vi "TestXYRobot.vi"() -> ()   [LabVIEW 2012]
uses:
  XY Stage/XYStage.llb/GlobalXYStage.vi
panel:
  in  "robot limits":T1={"xmin"=-16850, "xmax"=-1660, "ymin"=-15485, "ymax"=-550}
  in  "Home":bool
  out "XY Graph":cluster{"Y":dbl[], "Y":dbl[]}[](graph)=[{"Y"=[-1660.0, -16850.0, -16850.0, -1660.0, -1660.0], "Y"=[-550.0, -550.0, -15485.0, -15485.0, -550.0]}]
  in  "plot buffer":i32=5
  in  "Motor acc":i32=500
  in  "Motor low speed":i32=100
  in  "Motor high speed":i32=5000
  in  "Robot Position":T2(radio)
  in  "stop":bool
  out "Y position":i32=-550
  out "X position":i32=-1660
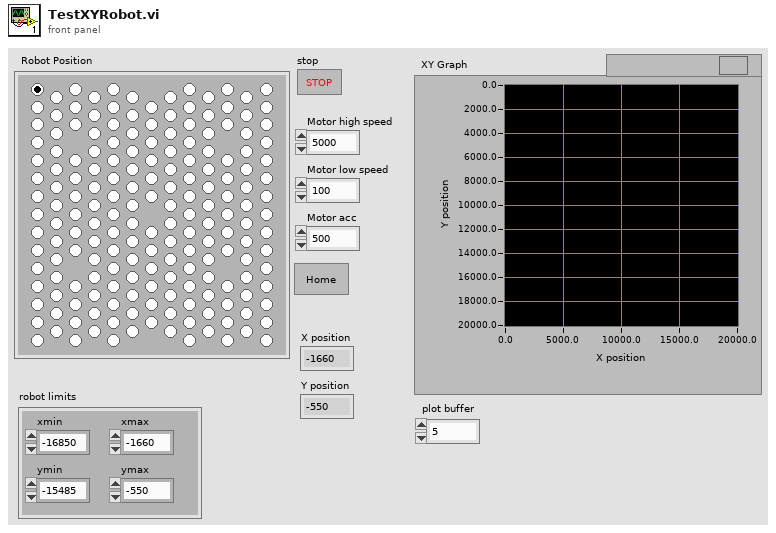
[diagram p1: front panel]
types:
  T1 = cluster{"xmin":i32, "xmax":i32, "ymin":i32, "ymax":i32}
  T2 = enum32{"Radio Selection 1", "Radio Selection 2", "Radio Selection 3", "Radio Selection 5", "Radio Selection 6", "Radio Selection 8", "Radio Selection 13", "Radio Selection 14", "Radio Selection 15", "Radio Selection 16", "Radio Selection 17", "Radio Selection 18", "Radio Selection 7", "Radio Selection 9", "Radio Selection 10", "Radio Selection 11", "Radio Selection 12", "Radio Selection 19", "Radio Selection 20", "Radio Selection 21", "Radio Selection 22", "Radio Selection 23", "Radio Selection 24", "Radio Selection 25", "Radio Selection 26", "Radio Selection 27", "Radio Selection 28", "Radio Selection 29", "Radio Selection 30", "Radio Selection 31", "Radio Selection 32", "Radio Selection 33", "Radio Selection 34", "Radio Selection 35", "Radio Selection 36", "Radio Selection 37", "Radio Selection 38", "Radio Selection 39", "Radio Selection 40", "Radio Selection 42", "Radio Selection 43", "Radio Selection 44", "Radio Selection 46", "Radio Selection 41", "Radio Selection 45", "Radio Selection 47", "Radio Selection 48", "Radio Selection 49", "Radio Selection 50", "Radio Selection 51", "Radio Selection 52", "Radio Selection 53", "Radio Selection 54", "Radio Selection 55", "Radio Selection 56", "Radio Selection 57", "Radio Selection 58", "Radio Selection 59", "Radio Selection 60", "Radio Selection 61", "Radio Selection 62", "Radio Selection 63", "Radio Selection 64", "Radio Selection 65", "Radio Selection 66", "Radio Selection 67", "Radio Selection 68", "Radio Selection 69", "Radio Selection 70", "Radio Selection 71", "Radio Selection 72", "Radio Selection 73", "Radio Selection 74", "Radio Selection 75", "Radio Selection 76", "Radio Selection 77", "Radio Selection 78", "Radio Selection 79", "Radio Selection 80", "Radio Selection 81", "Radio Selection 82", "Radio Selection 83", "Radio Selection 84", "Radio Selection 85", "Radio Selection 86", "Radio Selection 87", "Radio Selection 88", "Radio Selection 89", "Radio Selection 4", "Radio Selection 90", "Radio Selection 91", "Radio Selection 92", "Radio Selection 93", "Radio Selection 94", "Radio Selection 95", "Radio Selection 96", "Radio Selection 97", "Radio Selection 98", "Radio Selection 99", "Radio Selection 100", "Radio Selection 101", "Radio Selection 102", "Radio Selection 103", "Radio Selection 104", "Radio Selection 105", "Radio Selection 106", "Radio Selection 107", "Radio Selection 108", "Radio Selection 109", "Radio Selection 110", "Radio Selection 111", "Radio Selection 112", "Radio Selection 113", "Radio Selection 114", "Radio Selection 115", "Radio Selection 116", "Radio Selection 117", "Radio Selection 118", "Radio Selection 119", "Radio Selection 120", "Radio Selection 121", "Radio Selection 122", "Radio Selection 123", "Radio Selection 124", "Radio Selection 125", "Radio Selection 126", "Radio Selection 127", "Radio Selection 128", "Radio Selection 129", "Radio Selection 130", "Radio Selection 131", "Radio Selection 132", "Radio Selection 133", "Radio Selection 134", "Radio Selection 135", "Radio Selection 136", "Radio Selection 137", "Radio Selection 138", "Radio Selection 139", "Radio Selection 140", "Radio Selection 141", "Radio Selection 142", "Radio Selection 143", "Radio Selection 144", "Radio Selection 145", "Radio Selection 146", "Radio Selection 147", "Radio Selection 148", "Radio Selection 149", "Radio Selection 150", "Radio Selection 151", "Radio Selection 152", "Radio Selection 153", "Radio Selection 154", "Radio Selection 155", "Radio Selection 156", "Radio Selection 157", "Radio Selection 158", "Radio Selection 159", "Radio Selection 160", "Radio Selection 161", "Radio Selection 162", "Radio Selection 163", "Radio Selection 164", "Radio Selection 165", "Radio Selection 166", "Radio Selection 167", "Radio Selection 168", "Radio Selection 169", "Radio Selection 170", "Radio Selection 171", "Radio Selection 172", "Radio Selection 173", "Radio Selection 174", "Radio Selection 175", "Radio Selection 176", "Radio Selection 177", "Radio Selection 178", "Radio Selection 179", "Radio Selection 180", "Radio Selection 181", "Radio Selection 182"}
  T3 = enum8{"Enabled", "Disabled", "Disabled and Grayed Out"}
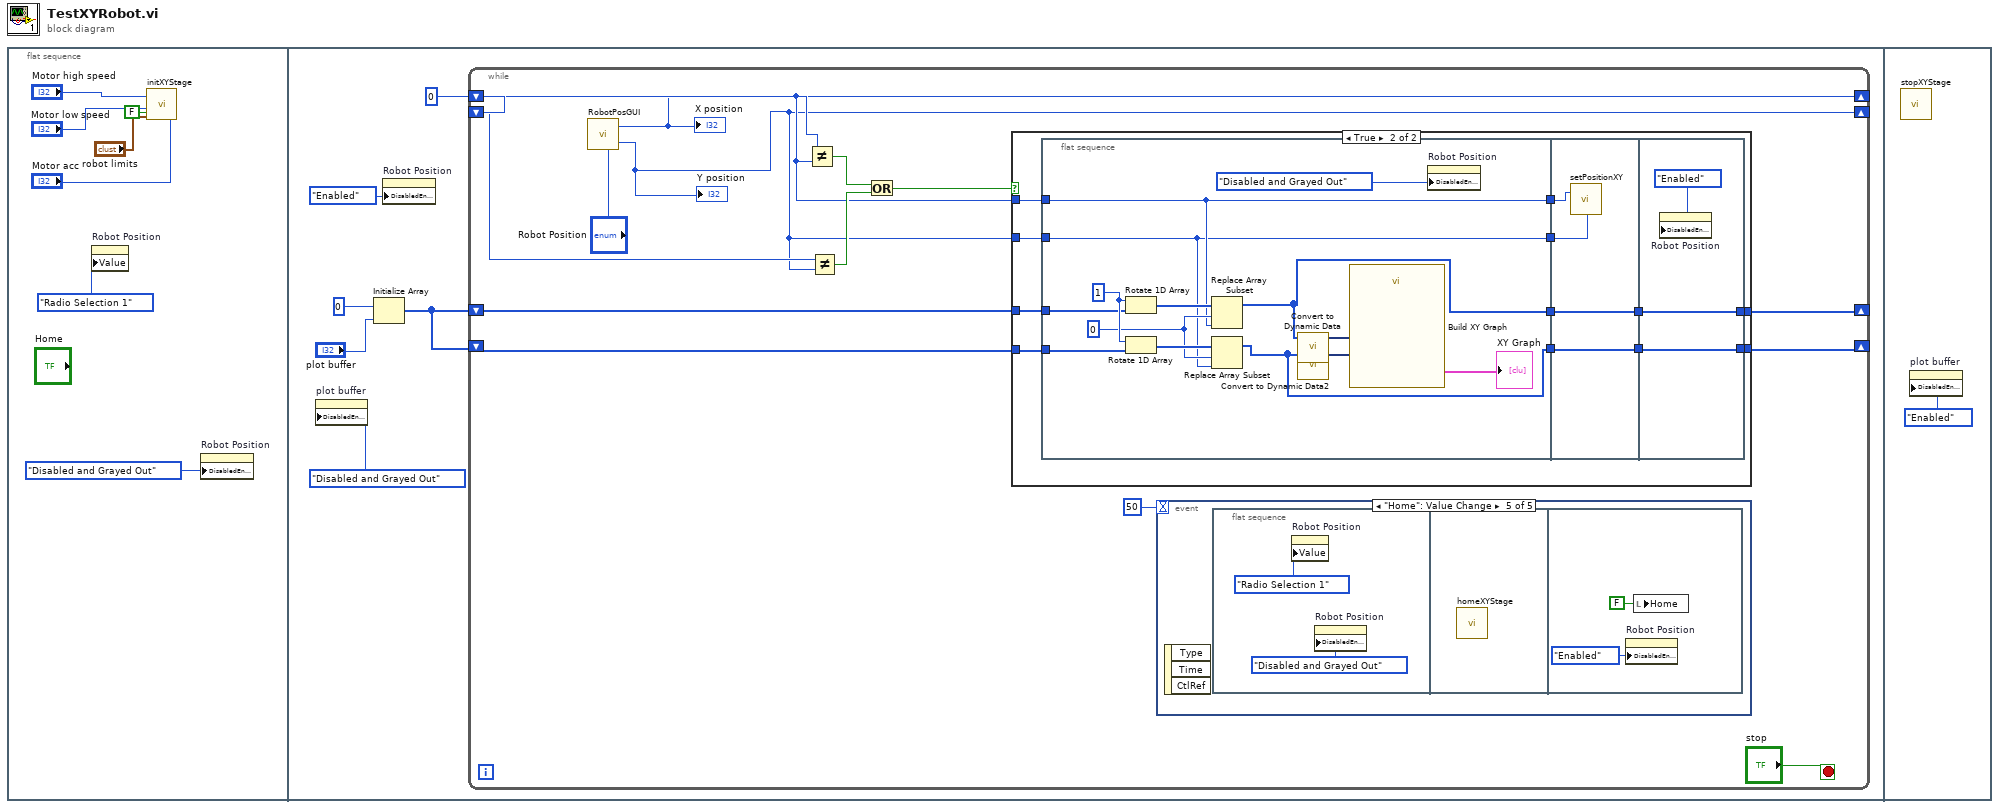
[diagram p0: block diagram]
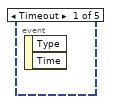
[diagram p2: hidden frame]
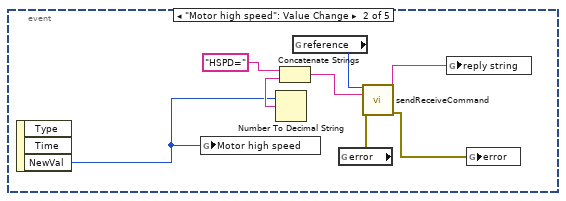
[diagram p3: hidden frame]
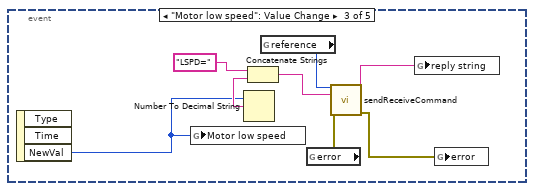
[diagram p4: hidden frame]
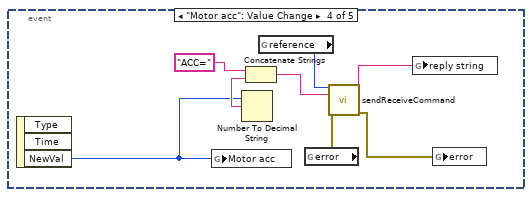
[diagram p5: hidden frame]
diagram:
  n1 = flat-sequence {
    frame #0 {
      n2 = property on="Robot Position" class="RadioBtnsControl (strict)"("Value"=T2."Radio Selection 1" ("Robot Position")) -> ()  [unwired: 2 in, 2 out]
      n3 = call "initXYStage.vi"("Motor high speed"="Motor high speed", "restart from\ncurrent position"=FALSE ("restart from\ncurrent position"), "Motor acc"="Motor acc", "Motor low speed"="Motor low speed", "robot limits"="robot limits") -> ()  [unwired: 1 out]
      n4 = property on="Robot Position" class="RadioBtnsControl (strict)"("DisabledEnum"=T3."Disabled and Grayed Out" ("Disabled")) -> ()  [unwired: 2 in, 2 out]
    }
    frame #1 {
      w13 = u16 0 ("X position")
      n5 = property on="plot buffer" class="DigNum (strict)"("DisabledEnum"=T3."Disabled and Grayed Out" ("Disabled")) -> ()  [unwired: 2 in, 2 out]
      n6 = Initialize Array(0 ("index"), "plot buffer") -> (w9:i32[])
      n7 = property on="Robot Position" class="RadioBtnsControl (strict)"("DisabledEnum"=T3."Enabled" ("Disabled")) -> ()  [unwired: 2 in, 2 out]
      n8 = while {
        shift-right: [w19] -> _
        shift-left: w13 -> [w25]
        shift-right: [w18] -> _
        shift-left: w13 -> [w24]
        shift-right: [w15] -> _
        shift-left: w9 -> [w17]
        shift-right: [w14] -> _
        shift-left: w9 -> [w16]
        stop <- "stop" stop-if-true
        n9 = call "RobotPosGUI.vi"("Robot Position"="Robot Position") -> ("X position"=w19:i32, "Y position"=w18:i32)  [unwired: 4 in]
        "X position" <- w19
        "Y position" <- w18
        n10 = Not Equal?(x=w25, y=w19) -> (x != y?=w22:bool)
        n11 = Not Equal?(x=w24, y=w18) -> (x != y?=w21:bool)
        n12 = Or(x=w22, y=w21) -> (x .or. y?=w20:bool)
        n13 = case shown="True" w20 {
          tunnel: w19 -> [_ w67]
          tunnel: w18 -> [_ w65]
          tunnel: w17 -> [w57 w69]
          tunnel: w16 -> [w56 w68]
          tunnel: [w57 w61] -> w15
          tunnel: [w56 w58] -> w14
          frame False {
          }
          frame True {
            n14 = flat-sequence {
              tunnel: w69 -> [w76]
              tunnel: w68 -> [w75]
              tunnel: w67 -> [w73]
              tunnel: [w73] -> w66
              tunnel: w65 -> [w72]
              tunnel: [w72] -> w64
              tunnel: [w71] -> w63
              tunnel: [w70] -> w60
              tunnel: w66 -> [w87]
              tunnel: w64 -> [w86]
              tunnel: w63 -> [w85]
              tunnel: [w85] -> w62
              tunnel: w60 -> [w84]
              tunnel: [w84] -> w59
              tunnel: w62 -> [w89]
              tunnel: [w89] -> w61
              tunnel: w59 -> [w88]
              tunnel: [w88] -> w58
              frame #0 {
                w77 = 1 ("n")
                w74 = 0 ("index")
                n15 = Rotate 1D Array(1:w76, 2:w77) -> (0:w79:i32[])
                n16 = Rotate 1D Array(1:w75, 2:w77) -> (0:w78:i32[])
                n17 = Replace Array Subset(array=w79, new element=w73, index=w74) -> (w71:i32[])
                n18 = Replace Array Subset(array=w78, new element=w72, index=w74) -> (w70:i32[])
                n19 = call "Convert to Dynamic Data"("Array"=w71) -> ("Dynamic Data Type"=w81:dynamicdata)  [unwired: 3 in]
                n20 = call "Convert to Dynamic Data2"("Array"=w70) -> ("Dynamic Data Type"=w80:dynamicdata)  [unwired: 3 in]
                n21 = call "Build XY Graph"("Y Input"=w80, "X Input"=w81) -> ("XY Graph"=→"XY Graph":cluster{"Y":dbl[], "Y":dbl[]}[])  [unwired: 3 in, 6 out]
                n22 = property on="Robot Position" class="RadioBtnsControl (strict)"("DisabledEnum"=T3."Disabled and Grayed Out" ("Disabled")) -> ()  [unwired: 2 in, 2 out]
              }
              frame #1 {
                n23 = call "setPositionXY.vi"("Y Position"=w86, "X Position"=w87) -> ()  [unwired: 1 in]
              }
              frame #2 {
                n24 = property on="Robot Position" class="RadioBtnsControl (strict)"("DisabledEnum"=T3."Enabled" ("Disabled")) -> ()  [unwired: 2 in, 2 out]
              }
            }
          }
        }
        n25 = event shown="[4] \"Home\": Value Change" {
          selector: _ -> [_ _ _ _ _]
          dyn-events: _ -> [_ _ _ _ _]
          timeout: 50 -> [_ _ _ _ _]
          event Timeout {
            n26 = event-data() -> ()  [unwired: 1 in, 2 out]
          }
          event "Motor high speed": Value Change {
            n27 = event-data() -> ("NewVal"=w28:i32)  [unwired: 1 in, 2 out]
            n28 = global write "GlobalXYStage.vi" "Motor high speed"(w28) -> ()
            n29 = Number To Decimal String(number=w28) -> (decimal integer string=w31:string)  [unwired: 1 in]
            n30 = Concatenate Strings("HSPD=" ("Axis"), w31) -> (w29:string)
            n31 = global read "GlobalXYStage.vi" "reference"() -> (w34:i32)
            n32 = global read "GlobalXYStage.vi" "error"() -> (w35:errorcluster)
            n33 = call "sendReceiveCommand.vi"("reference (in)"=w34, "write_string"=w29, "error in (no error)"=w35) -> ("read_string"=w33:string, "error out"=w32:errorcluster)  [unwired: 10 in, 1 out]
            n34 = global write "GlobalXYStage.vi" "reply string"(w33) -> ()
            n35 = global write "GlobalXYStage.vi" "error"(w32) -> ()
          }
          event "Motor low speed": Value Change {
            n36 = event-data() -> ("NewVal"=w36:i32)  [unwired: 1 in, 2 out]
            n37 = global write "GlobalXYStage.vi" "Motor low speed"(w36) -> ()
            n38 = Number To Decimal String(number=w36) -> (decimal integer string=w39:string)  [unwired: 1 in]
            n39 = Concatenate Strings("LSPD=" ("Axis"), w39) -> (w37:string)
            n40 = global read "GlobalXYStage.vi" "reference"() -> (w42:i32)
            n41 = global read "GlobalXYStage.vi" "error"() -> (w43:errorcluster)
            n42 = call "sendReceiveCommand.vi"("reference (in)"=w42, "write_string"=w37, "error in (no error)"=w43) -> ("read_string"=w41:string, "error out"=w40:errorcluster)  [unwired: 10 in, 1 out]
            n43 = global write "GlobalXYStage.vi" "reply string"(w41) -> ()
            n44 = global write "GlobalXYStage.vi" "error"(w40) -> ()
          }
          event "Motor acc": Value Change {
            n45 = event-data() -> ("NewVal"=w44:i32)  [unwired: 1 in, 2 out]
            n46 = global write "GlobalXYStage.vi" "Motor acc"(w44) -> ()
            n47 = Number To Decimal String(number=w44) -> (decimal integer string=w47:string)  [unwired: 1 in]
            n48 = Concatenate Strings("ACC=" ("Axis"), w47) -> (w45:string)
            n49 = global read "GlobalXYStage.vi" "reference"() -> (w50:i32)
            n50 = global read "GlobalXYStage.vi" "error"() -> (w51:errorcluster)
            n51 = call "sendReceiveCommand.vi"("reference (in)"=w50, "write_string"=w45, "error in (no error)"=w51) -> ("read_string"=w49:string, "error out"=w48:errorcluster)  [unwired: 10 in, 1 out]
            n52 = global write "GlobalXYStage.vi" "reply string"(w49) -> ()
            n53 = global write "GlobalXYStage.vi" "error"(w48) -> ()
          }
          event "Home": Value Change {
            n54 = event-data() -> ()  [unwired: 1 in, 3 out]
            n55 = flat-sequence {
              frame #0 {
                n56 = property on="Robot Position" class="RadioBtnsControl (strict)"("Value"=T2."Radio Selection 1" ("Robot Position")) -> ()  [unwired: 2 in, 2 out]
                n57 = property on="Robot Position" class="RadioBtnsControl (strict)"("DisabledEnum"=T3."Disabled and Grayed Out" ("Disabled")) -> ()  [unwired: 2 in, 2 out]
              }
              frame #1 {
                n58 = call "homeXYStage.vi"() -> ()  [unwired: 1 in]
              }
              frame #2 {
                n59 = property on="Robot Position" class="RadioBtnsControl (strict)"("DisabledEnum"=T3."Enabled" ("Disabled")) -> ()  [unwired: 2 in, 2 out]
                n60 = local write "Home"(FALSE ("Home")) -> ()
              }
            }
          }
        }
      }
    }
    frame #2 {
      n61 = call "stopXYStage.vi"() -> ()  [unwired: 12 in]
      n62 = property on="plot buffer" class="DigNum (strict)"("DisabledEnum"=T3."Enabled" ("Disabled")) -> ()  [unwired: 2 in, 2 out]
    }
  }
